vi "UART Read Byte Array.vi"(8 "Error In":errorcluster, 9 "Num Bytes":u8, 10 "UART Channel (0)":u8, 11 "LINX Resource":T1) -> (0 "Error Out":errorcluster, 2 "Data":u8[](array[numeric]), 3 "LINX Resource":T1)   [LabVIEW 2014, in "LMH-LINX.lvlib"]
doc: "Read the specified number of bytes from the specified UART channel's receive buffer as a byte array."
uses:
  <vilib>/MakerHub/LINX/LMH-LINX.lvlib
  <vilib>/MakerHub/LINX/Private/Type Defs/LINX Ref.ctl
  <vilib>/MakerHub/LINX/Private/Type Defs/Platform.ctl
  <vilib>/MakerHub/LINX/Private/Type Defs/Interface.ctl
  <vilib>/MakerHub/LINX/Private/Device/Type Defs/LINX Device Config.ctl
  <vilib>/MakerHub/LINX/Private/Device/Type Defs/TCP Config.ctl
  <vilib>/MakerHub/LINX/Private/Device/Type Defs/Channels.ctl
  <vilib>/MakerHub/LINX/Private/Type Defs/Peripheral.ctl
  <vilib>/MakerHub/LINX/Private/Utilties/Generate Error.vi
  <vilib>/MakerHub/LINX/Private/Device/Device.lvlib
  <vilib>/MakerHub/LINX/Private/Local IO/Local IO.lvlib
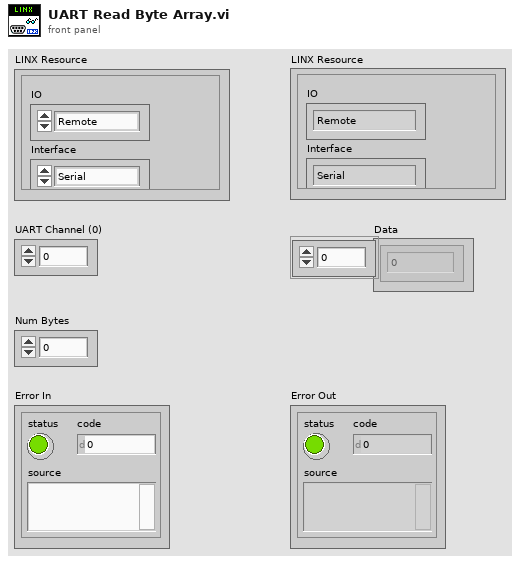
[diagram p1: front panel]
types:
  T1 = typedef "LMH-LINX.lvlib/LINX Ref.ctl" = cluster{"IO":T2, "Interface":T3, "LINX Device Config":T4}
  T2 = typedef "LMH-LINX.lvlib/Platform.ctl" = enum16{"Remote", "Local"}
  T3 = typedef "LMH-LINX.lvlib/Interface.ctl" = enum16{"Serial", "TCP"}
  T4 = typedef "LMH-LINX.lvlib/Device.lvlib/LINX Device Config.ctl" = cluster{"Interface":T3, "COM Port":refnum<visa-resource-name>, "TCP Configuration":T5, "Device Family":u8, "Device ID":u8, "Device Name":string, "TCP Ref":refnum<k5>, "Channels":T6}
  T5 = typedef "LMH-LINX.lvlib/Device.lvlib/TCP Config.ctl" = cluster{"IP Address":string, "Port":u16}
  T6 = typedef "LMH-LINX.lvlib/Channels.ctl" = cluster{"DI":u8[], "DO":u8[], "AI":u8[], "AO":u8[], "PWM":u8[], "QE":u8[], "UART":u8[], "I2C 2":u8[], "SPI":u8[], "CAN":u8[], "Servo":u8[], "AI Ref (V)":dbl, "AI Resolution (Bits)":u8, "AO Ref (V)":dbl, "AO Resolution (Bits)":u8}
  T7 = typedef "LMH-LINX.lvlib/Peripheral.ctl" = enum8{"DI", "DO", "AI", "AO", "PWM", "QE", "UART", "I2C", "SPI", "CAN", "Servo"}
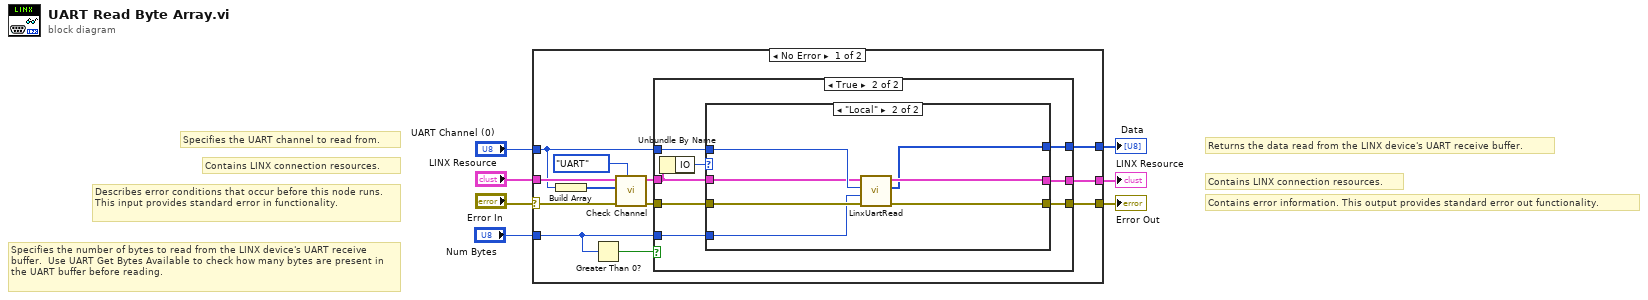
[diagram p0: block diagram]
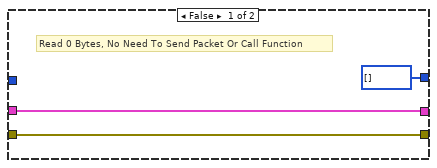
[diagram p2: hidden frame]
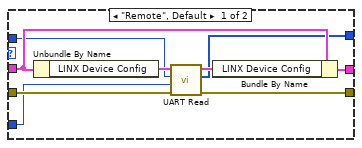
[diagram p3: hidden frame]
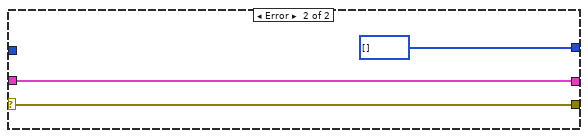
[diagram p4: hidden frame]
diagram:
  # "Specifies the number of bytes to read from the LINX device's UART receive buffer.  Use UART Get Bytes Available to check how many bytes are present in the UART buffer before reading."
  # "Specifies the UART channel to read from."
  # "Returns the data read from the LINX device's UART receive buffer."
  # "Contains LINX connection resources."
  # "Contains error information. This output provides standard error out functionality."
  # "Contains LINX connection resources."
  # "Describes error conditions that occur before this node runs. This input provides standard error in functionality."
  n1 = case shown="No Error" "Error In" {
    selector: "Error In" -> [w10 w49]
    tunnel: [w19 w49] -> w7
    tunnel: [w18 w48] -> w6
    tunnel: "LINX Resource" -> [w17 w48]
    tunnel: "UART Channel (0)" -> [w13 _]
    tunnel: "Num Bytes" -> [w8 _]
    tunnel: [w11 u8[] [] ("unsigned byte array")] -> w2
    frame No Error {
      n2 = Build Array(w13) -> (w14:u8[])
      n3 = Greater Than 0?(x=w8) -> (x > 0?=w9:bool)
      n4 = call <vilib>:"Check Channel.vi"("Peripheral"=Peripheral."UART", "Error In"=w10, "Channels"=w14, "LINX Resource"=w17) -> ("Error Out"=w15:errorcluster, "LINX Resource"=w16:T1)  [unwired: 5 in, 1 out]
      n5 = case shown="True" w9 {
        tunnel: [w20 w29] -> w19
        tunnel: [w21 w28] -> w18
        tunnel: w16 -> [w21 w27]
        tunnel: w15 -> [w20 w26]
        tunnel: w13 -> [_ w25]
        tunnel: w8 -> [_ w24]
        tunnel: [u8[] [] ("Data") w23] -> w11
        frame False {
          # "Read 0 Bytes, No Need To Send Packet Or Call Function"
        }
        frame True {
          n6 = Unbundle By Name(w27) -> ("IO"=w30:T2)
          n7 = case shown="\"Local\"" w30 {
            tunnel: w26 -> [w36 w46]
            tunnel: w27 -> [w39 w44]
            tunnel: [w37 w41] -> w29
            tunnel: [w38 w42] -> w28
            tunnel: w25 -> [w32 w45]
            tunnel: [w33 w40] -> w23
            tunnel: w24 -> [w31 w43]
            frame "Remote", Default {
              n8 = Unbundle By Name(w39) -> ("LINX Device Config"=w35:T4)
              n9 = call <vilib>:"UART Read.vi"("Error In"=w36, "Num Bytes"=w31, "UART Channel"=w32, "LINX Device Config"=w35) -> ("Error Out"=w37:errorcluster, "Data"=w33:u8[], "LINX Device Config"=w34:T4)  [unwired: 5 in]
              n10 = Bundle By Name(cluster=w39, "LINX Device Config"=w34) -> (w38:T1)
            }
            frame "Local" {
              n11 = call <vilib>:"LinxUartRead.vi"("Error In"=w46, "Num Bytes"=w43, "Uart Channel"=w45, "LINX Resource"=w44) -> ("Error Out"=w41:errorcluster, "Data"=w40:u8[], "LINX Resource"=w42:T1)  [unwired: 4 in, 1 out]
            }
          }
        }
      }
    }
    frame Error {
    }
  }
  "Error Out" <- w7
  "LINX Resource" <- w6
  "Data" <- w2
